vi "Hide Panel.vi"(8 "error in (no error)":errorcluster, 11 "Module ID":i32=-1) -> (0 "error out":errorcluster)   [LabVIEW 2015, in "Chat Window.lvlib"]
doc: "Send the Hide Panel request to the Module's Main.vi.\n_____\nBased on Delacor QMH Project Template 4.2.1.64."
uses:
  Chat Window.lvlib
  Hide Panel Argument--cluster.ctl
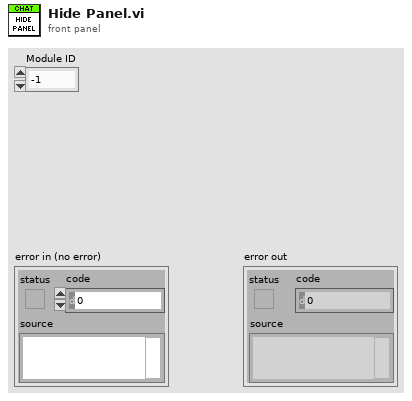
[diagram p1: front panel]
types:
  T1 = typedef "Chat Window.lvlib/Hide Panel Argument--cluster.ctl" = cluster{"Module ID":i32, "Hide Panel?":bool}
  T2 = typedef "Chat Window.lvlib/Request Events--cluster.ctl" = cluster{"Stop Module":refnum<user-event>, "Show Panel":refnum<user-event>, "Hide Panel":refnum<user-event>, "Show Diagram":refnum<user-event>, "Get Module Execution Status":refnum<user-event>, "New Message":refnum<user-event>, "Update Ring":refnum<user-event>}
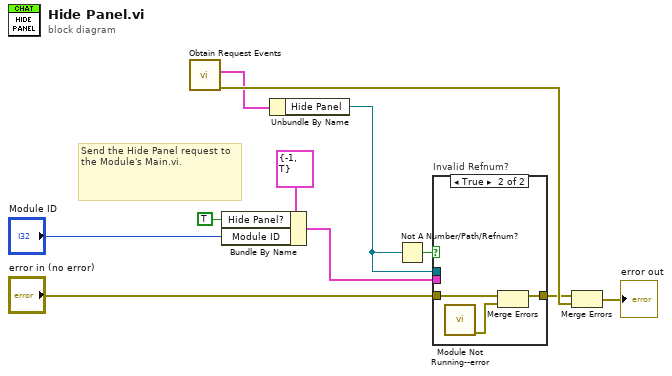
[diagram p0: block diagram]
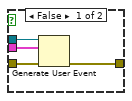
[diagram p2: hidden frame]
diagram:
  # "Send the Hide Panel request to the Module's Main.vi."
  n1 = call "Obtain Request Events.vi"() -> ("error out"=w10:errorcluster, "Chat Window Request Events"=w9:T2)  [unwired: 10 in]
  n2 = Bundle By Name(cluster=T1 {"Module ID"=-1, "Hide Panel?"=TRUE} ("Hide Panel Argument"), "Hide Panel?"=TRUE ("event data"), "Module ID"="Module ID") -> (w1:T1)
  n3 = Unbundle By Name(w9) -> ("Hide Panel"=w3:refnum<user-event>)
  n4 = Not A Number/Path/Refnum?(number/path/refnum=w3) -> (NaN/Path/Refnum?=w5:bool)
  n5 = case "Invalid Refnum?" shown="True" w5 {
    tunnel: "error in (no error)" -> [w15 w16]
    tunnel: [w14 w17] -> w4
    tunnel: w1 -> [w13 _]
    tunnel: w3 -> [w12 _]
    frame False {
      n6 = Generate User Event(user event=w12, event data cluster=w13, error in=w15) -> (error out=w14:errorcluster)  [unwired: 1 in, 1 out]
    }
    frame True {
      n7 = call "Module Not Running--error.vi"() -> ("error out"=w18:errorcluster)  [unwired: 11 in]
      n8 = Merge Errors(w16, w18) -> (w17:errorcluster)
    }
  }
  n9 = Merge Errors(w4, w10) -> (→"error out":errorcluster)
